vi "Read Bias Voltage String (V).vi"(11 "LCR-Measurement in":refnum<class "OTP_LCR_Meas.lvclass">) -> (2 "Bias Voltage String (V)":string="0:3/0.1,\n3:-3/0.1,\n-3:0/0.1", 3 "LCR-Measurement out":refnum<class "OTP_LCR_Meas.lvclass">)   [LabVIEW 2020, in "OTP_LCR_Meas.lvclass"]
uses:
  OTP_LCR_Meas.lvclass
  OTP_LCR_Meas.lvclass/OTP_LCR_Meas.ctl
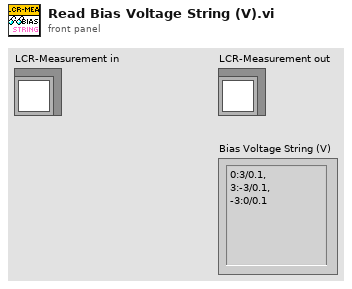
[diagram p1: front panel]
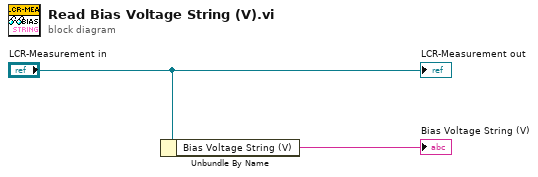
[diagram p0: block diagram]
diagram:
  n1 = Unbundle By Name("LCR-Measurement in") -> ("Bias Voltage String (V)"=→"Bias Voltage String (V)":string)
  "LCR-Measurement out" <- "LCR-Measurement in"
